vi "Read Units.vi"(8 "error in (no error)":errorcluster, 11 "Units in":refnum<class "Units.lvclass">) -> (0 "error out":errorcluster, 2 "Units":T1, 3 "Units out":refnum<class "Units.lvclass">)   [LabVIEW 2013, in "MaterialCharacterization.lvlib" / "Units.lvclass"]
uses:
  Units.lvclass
  ScanParser/Units.ctl
  Units.lvclass/Units.ctl
  ScanParser/MC-ScanParser.lvclass
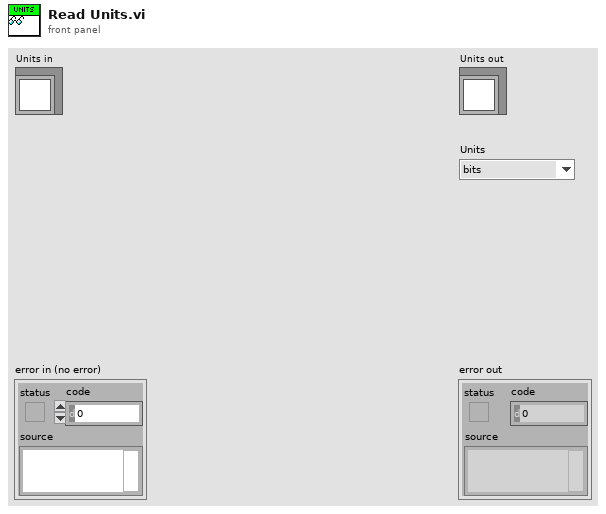
[diagram p1: front panel]
types:
  T1 = typedef "MaterialCharacterization.lvlib/MC-ScanParser.lvclass/Units.ctl" = enum16{"bits", "mm", "inch", "mils"}
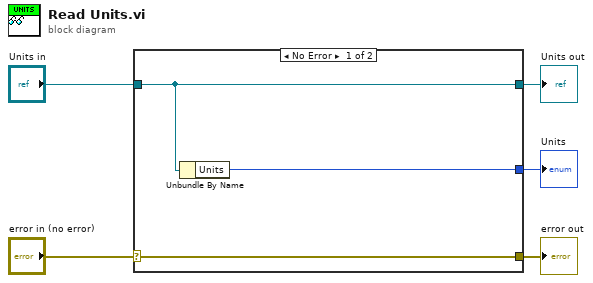
[diagram p0: block diagram]
diagram:
  n1 = case shown="No Error" "error in (no error)" {
    selector: "error in (no error)" -> [w8 w9]
    tunnel: [w8 w9] -> w4
    tunnel: [w7 w10] -> w2
    tunnel: "Units in" -> [w7 w10]
    tunnel: [w6 _] -> w1
    frame No Error {
      n2 = Unbundle By Name(w7) -> ("Units"=w6:T1)
    }
    frame Error {
    }
  }
  "error out" <- w4
  "Units out" <- w2
  "Units" <- w1
